vi "05b-multiple_functions.vi"() -> ()   [LabVIEW 2018, in "LV-0mq-Julia_roundtrip-lib.lvlib"]
uses:
  LV-0mq-Julia_roundtrip-lib.lvlib
  Server or client state.ctl
  detailed error info.ctl
  StackFrame.ctl
  Commands.ctl
  b50b62fa-0ed7-4d6a-8a9d-aa54acf293b0.vi
  b50b62fa-0ed7-4d6a-8a9d-aa54acf293b0.vi/b2054709-4ea8-4034-83b9-083b05da32b5.vi
  b50b62fa-0ed7-4d6a-8a9d-aa54acf293b0.vi/b2054709-4ea8-4034-83b9-083b05da32b5.vi/28a74c0b-3858-4202-956e-40757c91f57c.vi
  b50b62fa-0ed7-4d6a-8a9d-aa54acf293b0.vi/b2054709-4ea8-4034-83b9-083b05da32b5.vi/bfdf969c-92de-4c0b-a9f3-29470f9dac25.vi
  b50b62fa-0ed7-4d6a-8a9d-aa54acf293b0.vi/b2054709-4ea8-4034-83b9-083b05da32b5.vi/609f77b0-b2fe-4ab1-bf0c-f08ab84abc78.vi
  jl-scripts path.vi
  check ID validity.vi
  bindata_descr to JSON.vi
  check cluster field names.vi
  concat JSON.vi
  build request.vi
  Parse server response.vi
  log jl exceptions.vi
panel:
  in  "operation":u16(ring)
  in  "operands":cluster{"x":dbl, "y":dbl}={"x"=2.0, "y"=2.0}
  in  "next":bool
  out "x+y":dbl=nan
  out "detailed error info":T1
  out "current error":errorcluster
  out "final error":errorcluster
  out "short err code":u8
  in  "stop":bool
  out "ZMQ timeout":bool
  out "Julia script file path":path
  out "temporary script path":path
  out "Jl Server state":T3
  # "available functions loaded on start from the Julia server"
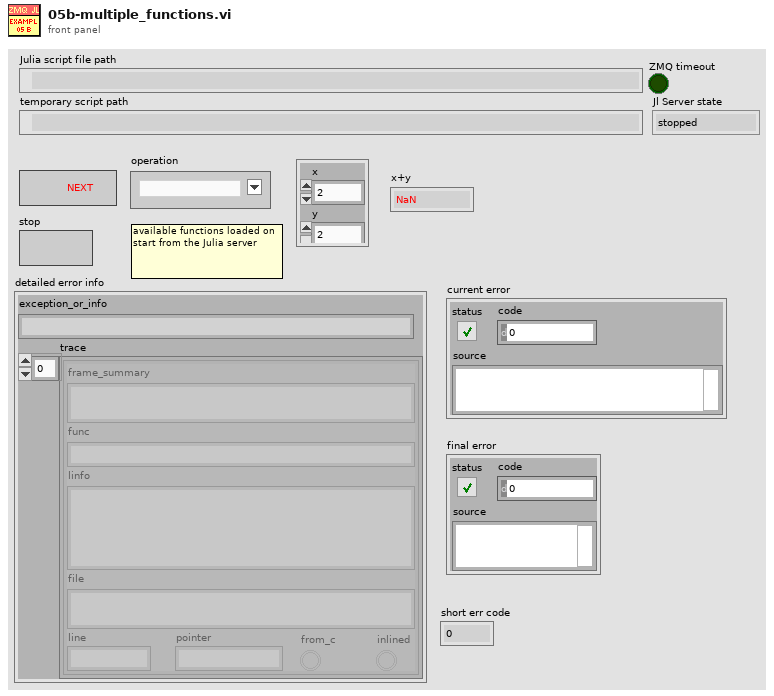
[diagram p1: front panel]
types:
  T1 = typedef "LV-0mq-Julia_roundtrip-lib.lvlib/detailed error info.ctl" = cluster{"exception_or_info":string, "trace":T2[]}
  T2 = typedef "LV-0mq-Julia_roundtrip-lib.lvlib/StackFrame.ctl" = cluster{"frame_summary":string, "func":string, "linfo":string, "file":string, "line":i32, "pointer":u64, "from_c":bool, "inlined":bool}
  T3 = typedef "LV-0mq-Julia_roundtrip-lib.lvlib/Server or client state.ctl" = enum16{"stopped", "running", "unknown"}
  T4 = typedef "LV-0mq-Julia_roundtrip-lib.lvlib/Commands.ctl" = enum16{"Start Jl-server & Init LV-client", "Send request & Get response ", "Stop Jl-server & Cleanup LV-client", "Cleanup LV-client", "Start Jl-server", "Stop Jl-server", "Init LV-Client", "Cleanup LV-Client", "(not allowed)", "Set LV Client state", "Set Jl Server state", "set ZMQ timeout", "read ZMQ timeout", "read-out state"}
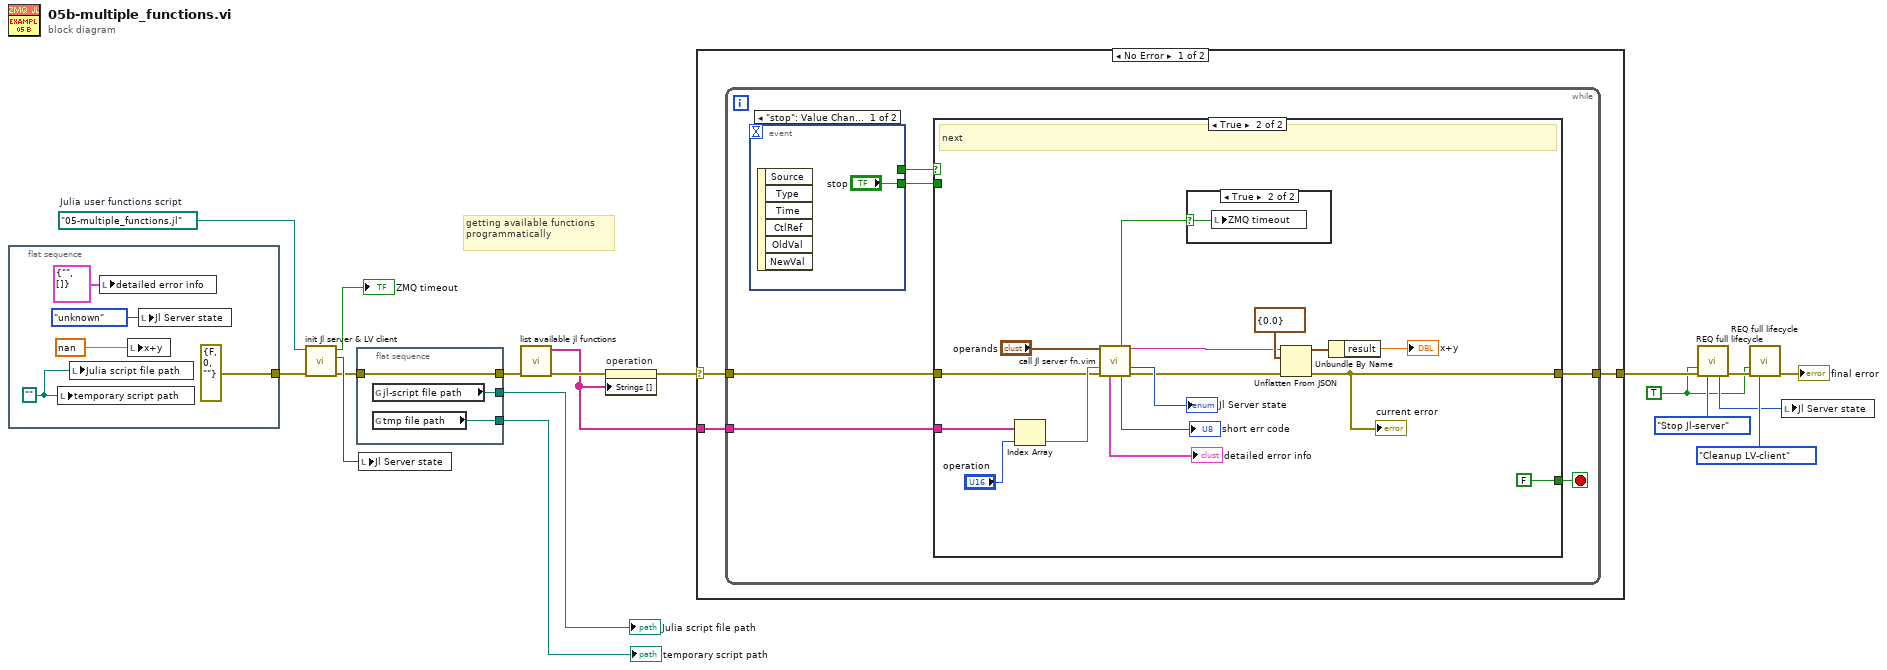
[diagram p0: block diagram]
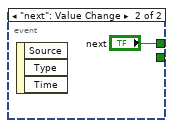
[diagram p2: hidden frame]
diagram:
  w5 = path "05-multiple_functions.jl"  # Julia user functions script
  w10 = TRUE ("Force command")
  # "getting available functions programmatically"
  n1 = flat-sequence {
    tunnel: [errorcluster {"status"=FALSE, "code"=0, "source"=""} ("error in (no error)")] -> w4
    frame #0 {
      w19 = path ""
      n2 = local write "temporary script path"(w19) -> ()
      n3 = local write "Julia script file path"(w19) -> ()
      n4 = local write "detailed error info"(T1 {"exception_or_info"="", "trace"=[]} ("detailed error info")) -> ()
      n5 = local write "x+y"(nan ("Server response")) -> ()
      n6 = local write "Jl Server state"(Server_or_client_state."unknown" ("Jl Server state out")) -> ()
    }
  }
  n7 = call "init Jl server & LV client.vi"("error in (no error)"=w4, "Julia user functions script"=w5) -> ("error out"=w1:errorcluster, "Jl Server state out"=w2:T3, "timeout?"=→"ZMQ timeout":bool)  [unwired: 7 in]
  n8 = flat-sequence {
    tunnel: [w26] -> w9
    tunnel: w1 -> [w26]
    tunnel: [w25] -> w12
    tunnel: [w24] -> w13
    frame #0 {
      n9 = global read "jl-scripts path.vi" "jl-script file path"() -> (w25:path)
      n10 = global read "jl-scripts path.vi" "tmp file path"() -> (w24:path)
    }
  }
  n11 = local write "Jl Server state"(w2) -> ()
  n12 = call "list available jl functions.vi"("error in (no error)"=w9) -> ("error out"=w8:errorcluster, "ext_fns"=w6:string[])  [unwired: 5 in, 4 out]
  n13 = property on="operation" class="Ring (strict)"(error in=w8, "Strings []"=w6) -> (error out=w7:errorcluster)  [unwired: 1 in, 1 out]
  n14 = case shown="No Error" w7 {
    selector: w7 -> [w28 w57]
    tunnel: [w29 w57] -> w18
    tunnel: w6 -> [w27 _]
    frame No Error {
      n15 = while {
        tunnel: w28 -> [w34]
        tunnel: [w35] -> w29
        tunnel: w27 -> [w30]
        stop <- w32 stop-if-true
        n16 = event shown="[0] \"stop\": Value Change" {
          selector: _ -> [_ _]
          dyn-events: _ -> [_ _]
          timeout: _ -> [_ _]
          tunnel: [_ "next"] -> w33
          tunnel: ["stop" _] -> w31
          event "stop": Value Change {
            n17 = event-data() -> ()  [unwired: 1 in, 6 out]
          }
          event "next": Value Change {
            n18 = event-data() -> ()  [unwired: 1 in, 3 out]
          }
        }
        n19 = case shown="True" w33 {
          tunnel: [w39 w52] -> w35
          tunnel: w34 -> [w39 w46]
          tunnel: [w38 FALSE ("stop this VI only")] -> w32
          tunnel: w31 -> [w38 _]
          tunnel: w30 -> [_ w50]
          frame False {
            # "stop"
          }
          frame True {
            # "next"
            n20 = Index Array(array=w50, index="operation") -> (element=w47:string)
            n21 = call "call Jl server fn.vim"("Arguments 1"="operands", "fun2call"=w47, "error in (no error)"=w46) -> ("timeout?"=w43:bool, "JSON received"=w41:string, "Jl Server state out"=→"Jl Server state":T3, "detailed error info"=→"detailed error info":T1, "return code"=→"short err code":u8, "error out"=w44:errorcluster)  [unwired: 6 in, 1 out]
            n22 = case shown="True" w43 {
              selector: w43 -> [_ w56]
              frame False {
              }
              frame True {
                n23 = local write "ZMQ timeout"(w56) -> ()
              }
            }
            n24 = Unflatten From JSON(JSON string=w41, type and defaults=cluster{"result":dbl} {"result"=0.0} ("parsed response"), error in (no error)=w44) -> (value=w54:cluster{"result":dbl}, error out=w52:errorcluster)  [unwired: 4 in]
            "current error" <- w52
            n25 = Unbundle By Name(w54) -> ("result"=→"x+y":dbl)
          }
        }
      }
    }
    frame Error {
    }
  }
  n26 = call "REQ full lifecycle.vi"("Force command"=w10, "error in"=w18, "command"=Commands."Stop Jl-server") -> ("Jl Server state out"=w11:T3, "error out"=w16:errorcluster)  [unwired: 6 in, 5 out]
  n27 = call "REQ full lifecycle.vi"("Force command"=w10, "error in"=w16, "command"=Commands."Cleanup LV-client") -> ("error out"=→"final error":errorcluster)  [unwired: 6 in, 6 out]
  n28 = local write "Jl Server state"(w11) -> ()
  "temporary script path" <- w13
  "Julia script file path" <- w12
